vi "While_loop.vi"() -> ()   [LabVIEW 2021]
panel:
  in  "milliseconds delay":u32
  in  "Stop While Loop":bool
  out "That's a Tank":dbl(slide) scale=0.0..1000.0
  in  "Vertical Multipler":dbl(slide) scale=0.0..10.0
  out "Indicator":dbl
  in  "Controler":dbl
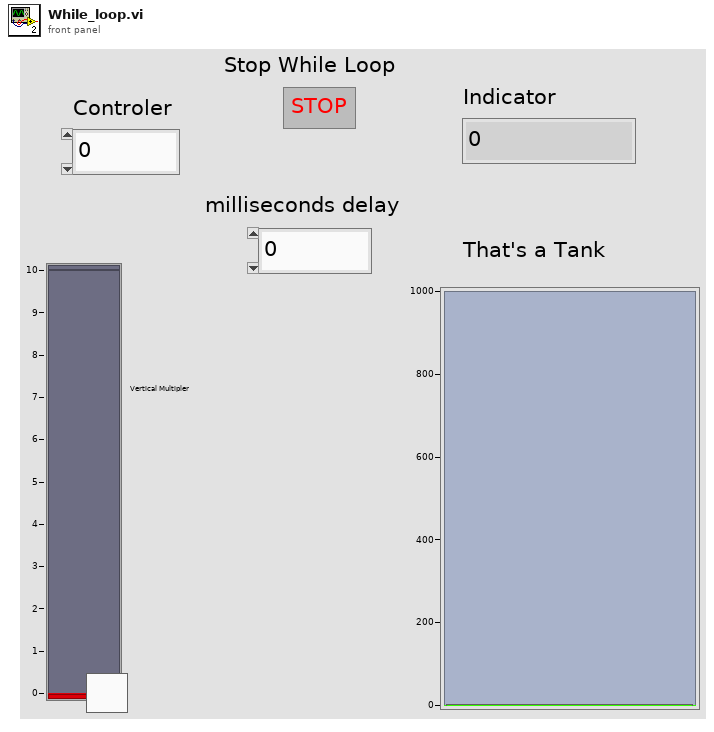
[diagram p1: front panel]
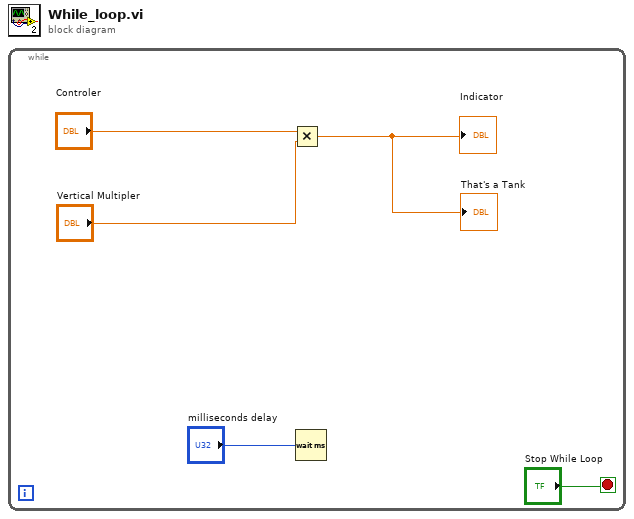
[diagram p0: block diagram]
diagram:
  n1 = while {
    stop <- "Stop While Loop" stop-if-true
    n2 = Multiply(x="Controler", y="Vertical Multipler") -> (x*y=→"Indicator" →"That's a Tank":dbl)
    n3 = Wait (ms)(milliseconds to wait="milliseconds delay") -> ()  [unwired: 1 out]
  }
